vi "FTW-ScheduledJobset-GetStatus.vi"(0 "FTW Scheduled Jobset":refnum<class "FTW-ScheduledJob.lvclass">[](array[class]), 5 "Identity":string, 11 "error in":errorcluster) -> (4 "FTW Scheduled Jobset out":refnum<class "FTW-ScheduledJob.lvclass">[](array[class]), 6 "Found?":bool, 15 "error out":errorcluster)   [LabVIEW 2015, in "FTW-ScheduledJob.lvclass"]
uses:
  FTW-ScheduledJob.lvclass
panel:
  out "Previous Scheduled Time":u32 format="%d msec"
  out "NextDeadline":u32 format="%d msec"
  # "Inputs"
  # "Outputs"
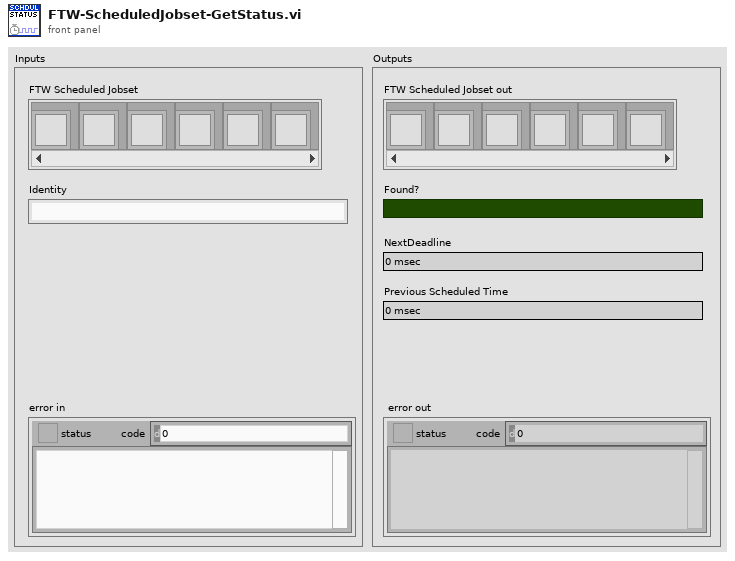
[diagram p1: front panel]
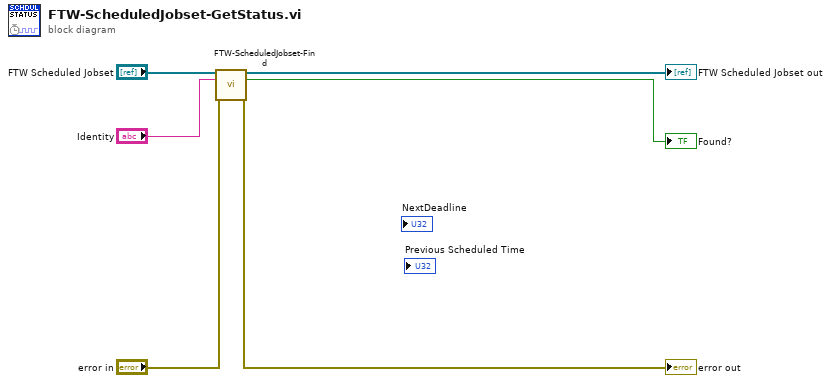
[diagram p0: block diagram]
diagram:
  n1 = call "FTW-ScheduledJobset-Find.vi"("FTW Scheduled Jobset"="FTW Scheduled Jobset", "Identity"="Identity", "error in"="error in") -> ("FTW Scheduled Jobset out"=→"FTW Scheduled Jobset out":refnum<class "FTW-ScheduledJob.lvclass">[], "Found?"=→"Found?":bool, "error out"=→"error out":errorcluster)  [unwired: 9 in, 1 out]
